vi "HW1_FPGA.vi"() -> ()   [LabVIEW 2019]
uses:
  <vilib>/rvi/Emulation/niFpgaGetClockAttributes.vi
  <vilib>/rvi/Emulation/niFpgaSctlEmulationGetInTimedLoop.vi
  <vilib>/rvi/Emulation/niFpgaEmulationReportErrorSimple.vi
  <vilib>/rvi/eio/common/nirviEmuTemplateMethod_errors.vi
  <vilib>/rvi/Emulation/niFpgaCriticalErrorInLSC.vi
  <vilib>/eio/EIONode/EIONode.xnode
panel:
  in  "Control  C/AO0":i16(knob) scale=0.0..5.0
  out "Indicator  C/AI1":i16
  in  "Stop":bool
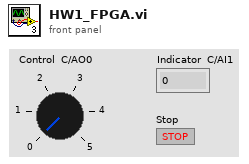
[diagram p1: front panel]
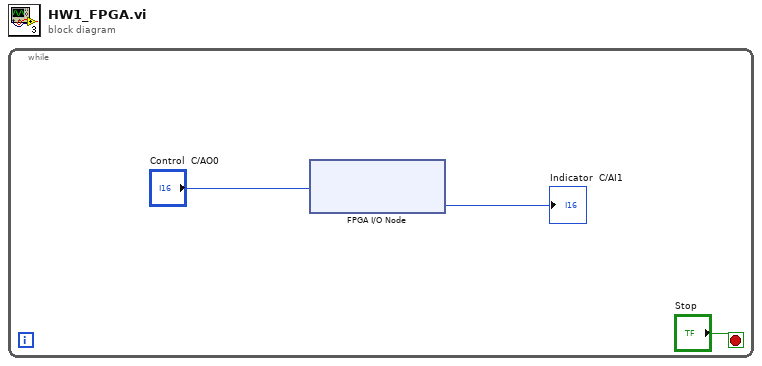
[diagram p0: block diagram]
diagram:
  n1 = while {
    stop <- "Stop" stop-if-true
    n2 = xnode "FPGA I/O Node"("ConnectorC/AO0"="Control  C/AO0") -> ("ConnectorC/AI1"=→"Indicator  C/AI1":i16)  [unwired: 2 in, 2 out]
  }
